vi "Gyro Change Mode.vi"(10 "DPS Mode":T1, 11 "I2CDevRef":T2 {"Device Address" format="%.0x"}) -> (3 "I2CDevRef Out":T2 {"Device Address" format="%.0x"})   [LabVIEW 2013]
uses:
  <vilib>/Rock Robotics/WPI/I2C/WPI_I2CDevRef.ctl
  <vilib>/Rock Robotics/SystemInterfaces/Typedef/FPGA_TypedefDigitalModule.ctl
  DPS Mode.ctl
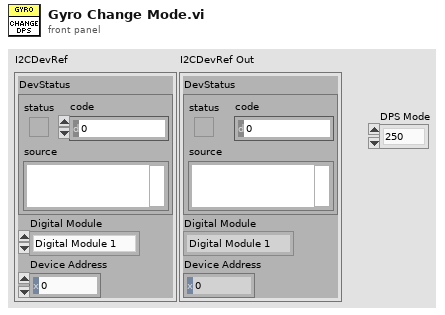
[diagram p1: front panel]
types:
  T1 = typedef "DPS Mode.ctl" = enum16{"250", "500", "2000"}
  T2 = typedef "WPI_I2CDevRef.ctl" = cluster{"DevStatus":errorcluster, "Digital Module":T3, "Device Address":u8}
  T3 = typedef "FPGA_TypedefDigitalModule.ctl" = enum16{"Digital Module 1", "Digital Module 2"}
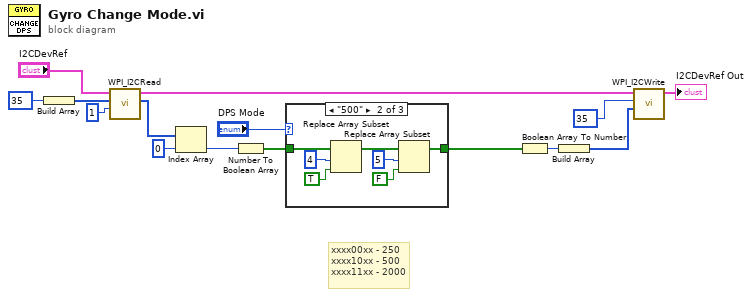
[diagram p0: block diagram]
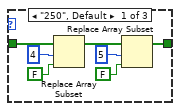
[diagram p2: hidden frame]
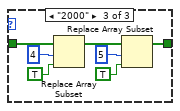
[diagram p3: hidden frame]
diagram:
  # "xxxx00xx - 250\nxxxx10xx - 500\nxxxx11xx - 2000"
  n1 = Build Array(u8 35 ("Data To Send")) -> (w6:u8[])
  n2 = call <vilib>:"WPI_I2CRead.vi"("I2CBytesToRead"=u8 1, "I2CRegister"=w6, "I2CDevRef"="I2CDevRef") -> ("Data Out"=w15:u8[], "I2CDevRef"=w10:T2)  [unwired: 6 in, 1 out]
  n3 = Index Array(array=w15, index=0) -> (element=w13:u8)
  n4 = Number To Boolean Array(number=w13) -> (Boolean array=w2:bool[])
  n5 = case shown="\"500\"" "DPS Mode" {
    tunnel: w2 -> [w18 w23 w30]
    tunnel: [w16 w24 w31] -> w1
    frame "250", Default {
      n6 = Replace Array Subset(array=w18, new element=FALSE ("new element/subarray"), index=4) -> (w17:bool[])
      n7 = Replace Array Subset(array=w17, new element=FALSE ("new element/subarray"), index=5) -> (w16:bool[])
    }
    frame "500" {
      n8 = Replace Array Subset(array=w23, new element=TRUE ("new element/subarray"), index=4) -> (w25:bool[])
      n9 = Replace Array Subset(array=w25, new element=FALSE ("new element/subarray"), index=5) -> (w24:bool[])
    }
    frame "2000" {
      n10 = Replace Array Subset(array=w30, new element=TRUE ("new element/subarray"), index=4) -> (w32:bool[])
      n11 = Replace Array Subset(array=w32, new element=TRUE ("new element/subarray"), index=5) -> (w31:bool[])
    }
  }
  n12 = Boolean Array To Number(Boolean array=w1) -> (number=w12:u32)
  n13 = Build Array(w12) -> (w11:u32[])
  n14 = call <vilib>:"WPI_I2CWrite.vi"("I2CDataToSend"=w11, "I2CRegister"=u8 35 ("Data To Send"), "I2CDevRef"=w10) -> ("I2CDevRef"=→"I2CDevRef Out":T2)  [unwired: 7 in, 1 out]
